vi "Get Child Types.vi"(8 "error in (no error)":errorcluster, 11 "LVClusterType.lvclass in":refnum<class "LVClusterType.lvclass">) -> (0 "error out":errorcluster, 2 "Children":refnum<class "LVType.lvclass">[](array[class]), 3 "LVClusterType.lvclass out":refnum<class "LVClusterType.lvclass">)   [LabVIEW 2020, in "LVDataTypes.lvlib" / "LVClusterType.lvclass"]
uses:
  <vilib>/AppBuilder/Engine/WebServiceDescription/LVDataTypes/LVClusterType/LVClusterType.lvclass
  <vilib>/AppBuilder/Engine/WebServiceDescription/LVDataTypes/LVType/LVType.lvclass
  <vilib>/AppBuilder/Engine/WebServiceDescription/LVDataTypes/LVClusterType/LVClusterType.lvclass/LVClusterType.ctl
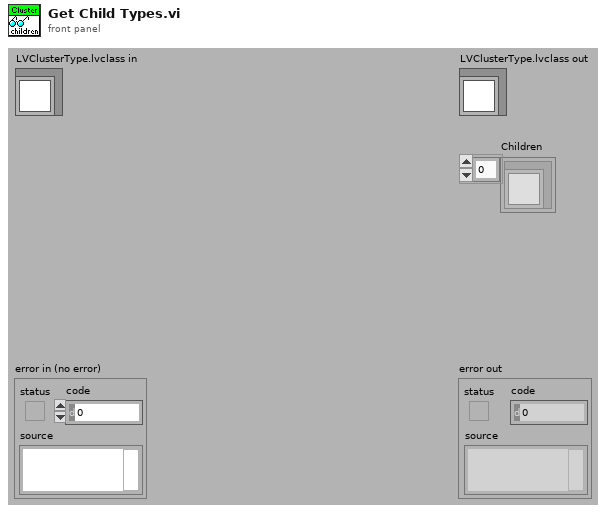
[diagram p1: front panel]
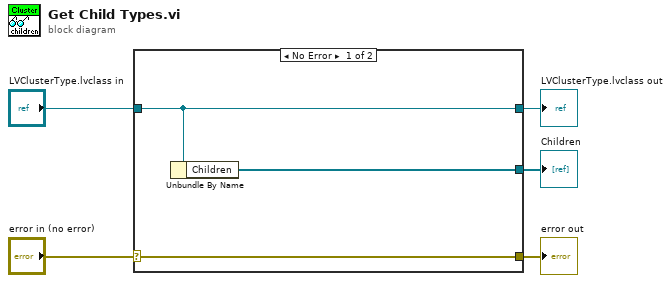
[diagram p0: block diagram]
diagram:
  n1 = case shown="No Error" "error in (no error)" {
    selector: "error in (no error)" -> [w8 w9]
    tunnel: [w8 w9] -> w4
    tunnel: [w7 w10] -> w2
    tunnel: "LVClusterType.lvclass in" -> [w7 w10]
    tunnel: [w6 _] -> w1
    frame No Error {
      n2 = Unbundle By Name(w7) -> ("Children"=w6:refnum<class "LVType.lvclass">[])
    }
    frame Error {
    }
  }
  "error out" <- w4
  "LVClusterType.lvclass out" <- w2
  "Children" <- w1
